vi "DO DAQ.vi"(11 "Queue ref":T1) -> ()   [LabVIEW 2022 SP3]
uses:
  Controls/All Queue.ctl
  Controls/DAQ case.ctl
  Controls/UI Data.ctl
  Controls/All Loop Status.ctl
  <vilib>/DAQmx/write.llb/DAQmx Write (Digital 1D Bool NChan 1Samp 1Line).vi
  Create Task/DO Create Task.vi
  Sub VI's/Global 1.vi
  <vilib>/DAQmx/miscellaneous.llb/DAQmx Fill In Error Info.vi
panel:
  out "x-y":u32
  # "TC channel list"
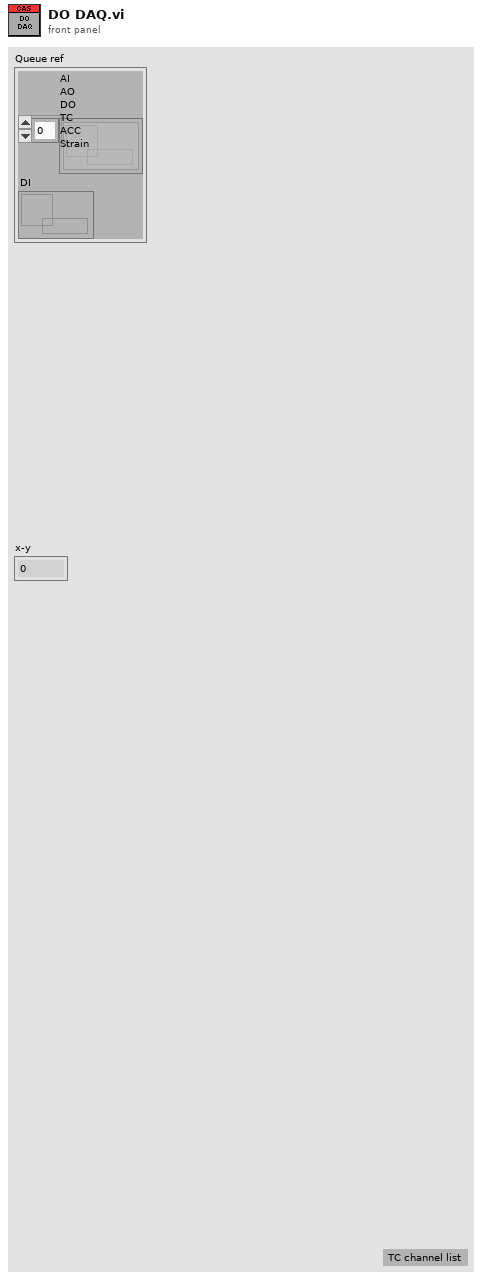
[diagram p1: front panel]
types:
  T1 = typedef "All Queue.ctl" = cluster{"AI\nAO\nDO\nTC\nACC\nStrain":refnum<queue>[], "DI":refnum<queue>}
  T2 = cluster{"in progress?":bool, "Start DAQ":refnum<notifier>, "UI Data":refnum<notifier>, "task out":refnum<k21>, "DO Ref":refnum<queue>, "Loop Rate":u32}
  T3 = typedef "DAQ case.ctl" = enum16{"Initailise", "Create Task", "Polevent", "Acquire", "Stop DAQ", "Error", "Exit"}
  T4 = typedef "All Loop Status.ctl" = enum16{"AI", "AO", "DI", "DO", "TC", "Strain", "ACC", "RT", "Log"}
  T5 = enum16{"Init", "Read 'All'", "Read 'n'", "Read '1'", "Write '1'", "Write 'n'", "Write 'All'"}
  T6 = typedef "All Notifer.ctl" = cluster{"UI Data":refnum<notifier>, "Start DAQ":refnum<notifier>, "Start Log":refnum<notifier>}
  T7 = cluster{"Analog input":bool, "Analog Output":bool, "Digital input":bool, "Digital output":bool, "Thermocouple":bool, "Strain Gauge":bool, "Accelerometer":bool}
  T8 = typedef "Config.ctl" = cluster{"AO config":cluster{"Channel_Name":string, "Channel_Number":string, "Default_Value":dbl, "Units":string}[], "AI config":cluster{"Channel_Name":string, "Channel_Number":string, "Pre_Scale_min":dbl, "Pre_Scale_max":dbl, "Sensor_min":dbl, "Sensor_max":dbl, "Units":string}[], "DI config":cluster{"Channel_Name":string, "Channel_Number":string, "Default_Value":bool, "DI invert?":bool}[], "DO config":cluster{"Channel_Name":string, "Channel_Number":string, "Default_Value":bool, "DO invert?":bool}[], "TC config":cluster{"Channel_Name":string, "Channel_Number":string, "Pre_Scale_min":dbl, "Pre_Scale_max":dbl, "units":i32, " type":i32}[], "ACC config":cluster{"Channel_Name":string, "Channel_Number":string, "Pre_Scale_min":dbl, "Pre_Scale_max":dbl, "Terminal configuration":i32, "Sensitivity":dbl, "Sensitivity units":i32}[], "SG config":cluster{"Channel_Name":string, "Channel_Number":string, "Pre_Scale_min":dbl, "Pre_Scale_max":dbl}[], "Strain Gauge Settings":cluster{"poisson ratio":dbl, "nominal gage resistance":dbl, "gage factor":dbl}, "bridge information":cluster{"strain configuration":i32, "lead wire resistance":dbl, "initial bridge voltage":dbl, "voltage excitation source":i32, "voltage excitation value":dbl}, "Sample Rate":cluster{"AI Sample Rate":dbl, "AO Sample Rate":dbl, "DI Sample Rate":dbl, "TC Sample Rate":dbl, "DO Sample Rate":dbl, "SG Sample Rate":dbl, "ACC Sample Rate":dbl}}
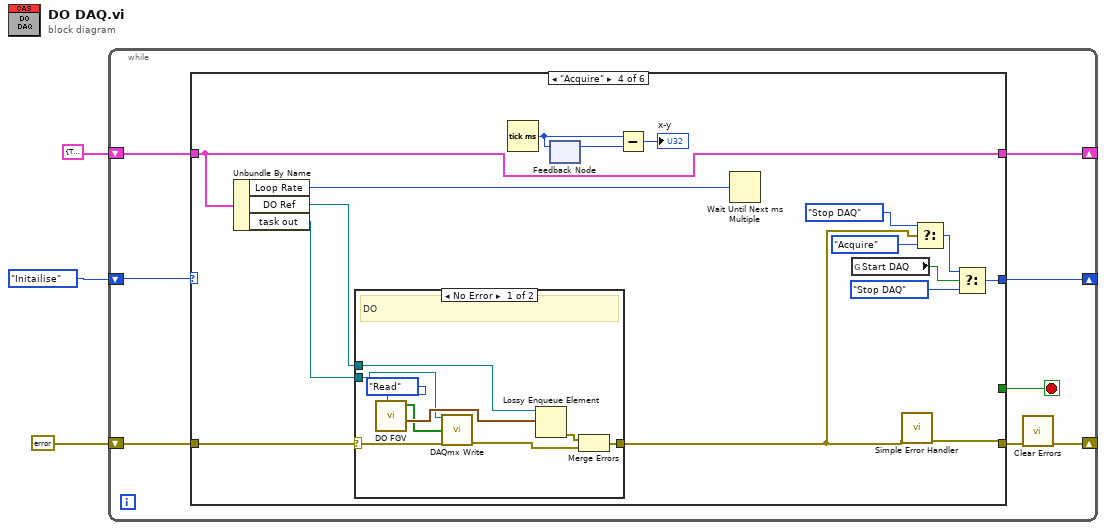
[diagram p0: block diagram]
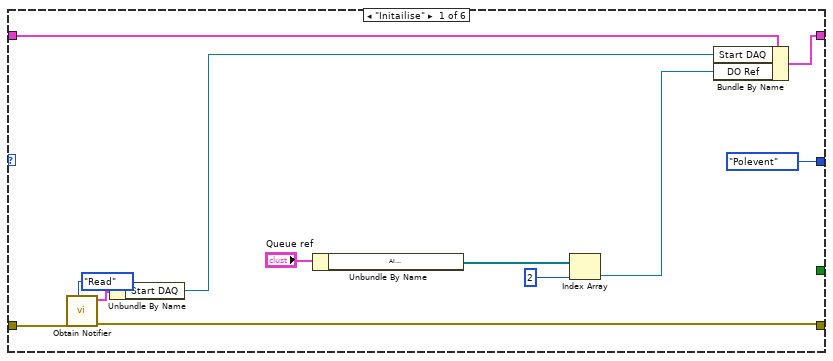
[diagram p2: hidden frame]
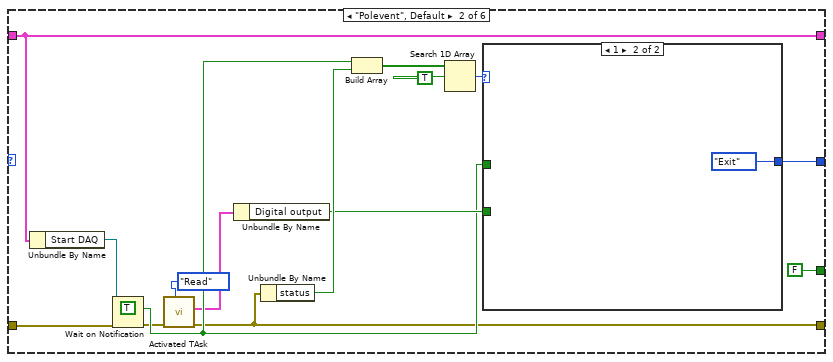
[diagram p3: hidden frame]
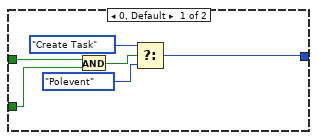
[diagram p4: hidden frame]
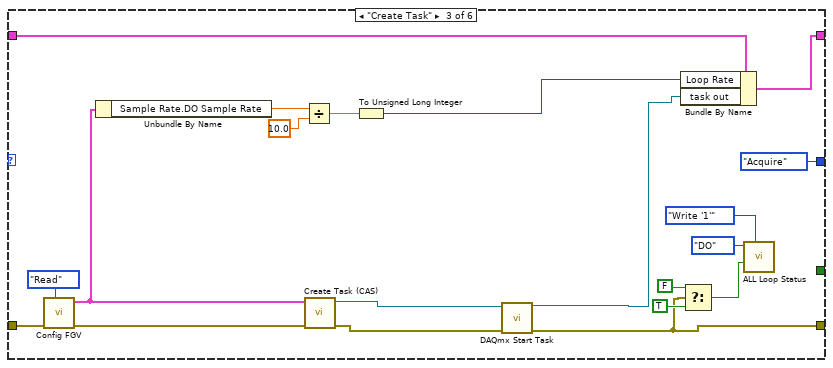
[diagram p5: hidden frame]
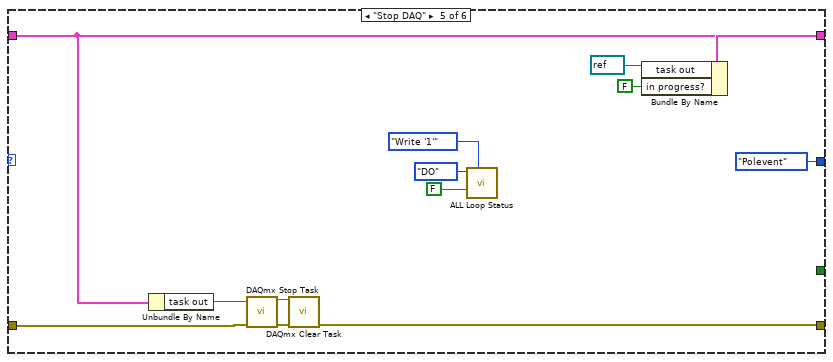
[diagram p7: hidden frame]
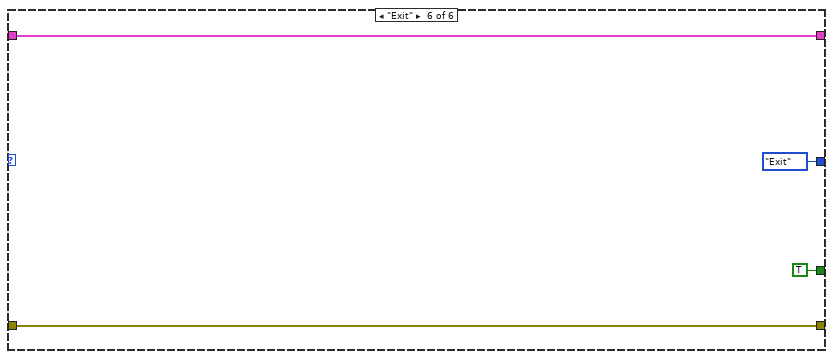
[diagram p8: hidden frame]
diagram:
  n1 = while {
    shift-right: [w4] -> _
    shift-left: errorcluster {"status"=FALSE, "code"=0, "source"=""} ("error out") -> [w10]
    shift-right: [w8] -> _
    shift-left: T2 {"in progress?"=TRUE, "Start DAQ"=refnum, "UI Data"=refnum, "task out"="", "DO Ref"=refnum, "Loop Rate"=0} -> [w9]
    shift-right: [w7] -> _
    shift-left: DAQ_case."Initailise" -> [w6]
    stop <- w11 stop-if-true
    n2 = case shown="\"Acquire\"" w6 {
      tunnel: [_ FALSE _ _ _ TRUE] -> w11
      tunnel: w10 -> [w22 w27 w63 w72 w97 w109]
      tunnel: [w21 w25 w50 w68 w98 w109] -> w5
      tunnel: w9 -> [w19 w37 w65 w73 w102 w108]
      tunnel: [w17 w37 w64 w73 w103 w108] -> w8
      tunnel: [DAQ_case."Polevent" w38 DAQ_case."Acquire" w74 DAQ_case."Polevent" DAQ_case."Exit"] -> w7
      frame "Initailise" {
        n3 = call "Obtain Notifier.vi"("Case"=enum16{"Obtain", "Read"}."Read", "error in (no error)"=w22) -> ("error out"=w21:errorcluster, "notifiers out"=w20:T6)  [unwired: 8 in]
        n4 = Unbundle By Name(w20) -> ("Start DAQ"=w18:refnum<notifier>)
        n5 = Unbundle By Name("Queue ref") -> ("AI\nAO\nDO\nTC\nACC\nStrain"=w14:refnum<queue>[])
        n6 = Index Array(array=w14, index=2) -> (element=w12:refnum<queue>)
        n7 = Bundle By Name(cluster=w19, "Start DAQ"=w18, "DO Ref"=w12) -> (w17:T2)
      }
      frame "Polevent", Default {
        n8 = Unbundle By Name(w37) -> ("Start DAQ"=w36:refnum<notifier>)
        n9 = Wait on Notification(notifier=w36, ignore previous (F)=TRUE, error in (no error)=w27) -> (notification=w28:bool, error out=w26:errorcluster)  [unwired: 1 in, 2 out]
        n10 = call "Activated TAsk.vi"("Enum"=enum16{"Read", "Write"}."Read", "error in (no error)"=w26) -> ("error out"=w25:errorcluster, "Activate Task 2"=w24:T7)  [unwired: 7 in, 1 out]
        n11 = Unbundle By Name(w24) -> ("Digital output"=w29:bool)
        n12 = Unbundle By Name(w25) -> ("status"=w35:bool)
        n13 = Build Array(w28, w35) -> (w33:bool[])
        n14 = Search 1D Array(1D array=w33, element=TRUE) -> (index of element=w31:i32)  [unwired: 1 in]
        n15 = case shown="1" w31 {
          tunnel: [w44 DAQ_case."Exit"] -> w38
          tunnel: w29 -> [w41 _]
          tunnel: w28 -> [w40 _]
          frame 0, Default {
            n16 = And(x=w40, y=w41) -> (x .and. y?=w42:bool)
            n17 = Select(t=DAQ_case."Create Task", s=w42, f=DAQ_case."Polevent") -> (s? t:f=w44:T3)
          }
          frame 1 {
          }
        }
      }
      frame "Create Task" {
        n18 = call "Config FGV.vi"("Enum"=enum16{"Read", "Write"}."Read", "error in (no error)"=w63) -> ("error out"=w61:errorcluster, "Data"=w55:T8)  [unwired: 8 in]
        n19 = Unbundle By Name(w55) -> ("Sample Rate.DO Sample Rate"=w54:dbl)
        n20 = Divide(x=w54, y=10.0) -> (x/y=w52:dbl)
        n21 = call-poly "Create Task (CAS).vi"("error in"=w61, "Data"=w55) -> ("error out"=w49:errorcluster, "task out"=w48:refnum<k21>)  [unwired: 7 in, 1 out]
        n22 = To Unsigned Long Integer(number=w52) -> (unsigned 32bit integer=w51:u32)
        n23 = call <vilib>:"DAQmx Start Task.vi"("task/channels in"=w48, "error in"=w49) -> ("task out"=w47:refnum<k21>, "error out"=w50:errorcluster)  [unwired: 12 in]
        n24 = Bundle By Name(cluster=w65, "Loop Rate"=w51, "task out"=w47) -> (w64:T2)
        n25 = Select(t=FALSE, s=w50, f=TRUE) -> (s? t:f=w58:bool)
        n26 = call "ALL Loop Status.vi"("Option"=T5."Write '1'", "Status"=w58, "Loop"=All_Loop_Status."DO") -> ()  [unwired: 6 in, 3 out]
      }
      frame "Acquire" {
        n27 = Unbundle By Name(w73) -> ("Loop Rate"=w67:u32, "DO Ref"=w71:refnum<queue>, "task out"=w70:refnum<k21>)
        n28 = case shown="No Error" w72 {
          selector: w72 -> [w89 w92]
          tunnel: w70 -> [w84 _]
          tunnel: [w90 w92] -> w69
          tunnel: w71 -> [w86 _]
          frame No Error {
            # "DO"
            n29 = call "DO FGV.vi"("Enum"=enum16{"Read", "Write", "Start time", "init"}."Read") -> ("DO Waveform"=w85:waveform(dbl)[], "DO out"=w83:bool[])  [unwired: 8 in, 1 out]
            n30 = call-poly <vilib>:"DAQmx Write.vi"("task/channels in"=w84, "data"=w83, "error in"=w89) -> ("error out"=w88:errorcluster)  [unwired: 10 in, 2 out]
            n31 = Lossy Enqueue Element(queue=w86, element=w85) -> (error out=w91:errorcluster)  [unwired: 1 in, 3 out]
            n32 = Merge Errors(w91, w88) -> (w90:errorcluster)
          }
          frame Error {
          }
        }
        n33 = Tick Count (ms)() -> (millisecond timer value=w82:u32)
        n34 = feedback-in #1(w82) -> ()
        n35 = feedback #1() -> (w81:u32)  [unwired: 1 in]
        n36 = Subtract(x=w82, y=w81) -> (x-y=→"x-y":u32)
        n37 = Wait Until Next ms Multiple(millisecond multiple=w67) -> ()  [unwired: 1 out]
        n38 = global read "Global 1.vi" "Start DAQ"() -> (w77:bool)
        n39 = call <vilib>:"Simple Error Handler.vi"("error in (no error)"=w69) -> ("error out"=w68:errorcluster)  [unwired: 4 in, 4 out]
        n40 = Select(t=DAQ_case."Stop DAQ", s=w69, f=DAQ_case."Acquire") -> (s? t:f=w76:T3)
        n41 = Select(t=w76, s=w77, f=DAQ_case."Stop DAQ") -> (s? t:f=w74:T3)
      }
      frame "Stop DAQ" {
        n42 = Unbundle By Name(w102) -> ("task out"=w96:refnum<k21>)
        n43 = call <vilib>:"DAQmx Stop Task.vi"("task/channels in"=w96, "error in"=w97) -> ("task out"=w95:refnum<k21>, "error out"=w99:errorcluster)  [unwired: 12 in]
        n44 = call <vilib>:"DAQmx Clear Task.vi"("task in"=w95, "error in"=w99) -> ("error out"=w98:errorcluster)  [unwired: 13 in]
        n45 = call "ALL Loop Status.vi"("Option"=T5."Write '1'", "Status"=FALSE, "Loop"=All_Loop_Status."DO") -> ()  [unwired: 6 in, 3 out]
        n46 = Bundle By Name(cluster=w102, "task out"=refnum<k21> refnum, "in progress?"=FALSE) -> (w103:T2)
      }
      frame "Exit" {
      }
    }
    n47 = call <vilib>:"Clear Errors.vi"("error in (no error)"=w5) -> ("error out"=w4:errorcluster)  [unwired: 5 in, 1 out]
  }
